vi "Read Write.vi"(8 "error in (no error)":errorcluster, 11 "File Observer in":refnum<class "File Observer.lvclass">) -> (0 "error out":errorcluster, 2 "Write":bool, 3 "File Observer out":refnum<class "File Observer.lvclass">)   [LabVIEW 2014, in "File Observer.lvclass"]
uses:
  File Observer.lvclass
  File Observer.lvclass/File Observer.ctl
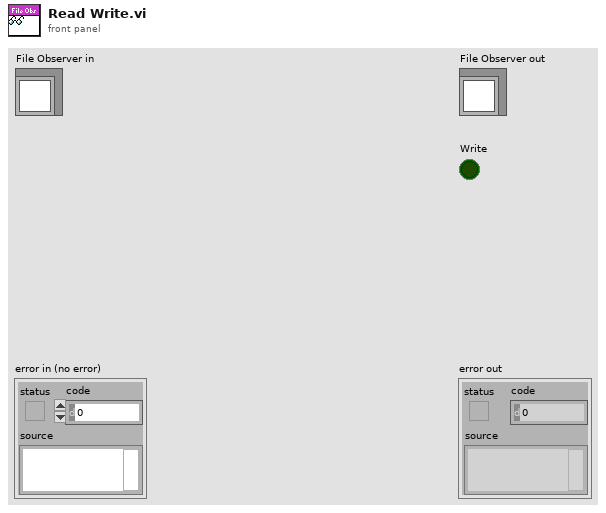
[diagram p1: front panel]
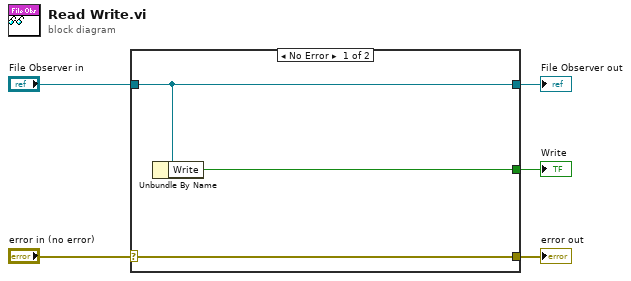
[diagram p0: block diagram]
diagram:
  n1 = case shown="No Error" "error in (no error)" {
    selector: "error in (no error)" -> [w8 w9]
    tunnel: [w8 w9] -> w4
    tunnel: [w7 w10] -> w2
    tunnel: "File Observer in" -> [w7 w10]
    tunnel: [w6 _] -> w1
    frame No Error {
      n2 = Unbundle By Name(w7) -> ("Write"=w6:bool)
    }
    frame Error {
    }
  }
  "error out" <- w4
  "File Observer out" <- w2
  "Write" <- w1
